vi "VNA Empty Driver Output.vi"() -> (0 "VNA Driver Output":T1 {"Parameters Measured"."Channel" min=1 max=99 step=1; "Parameters Measured"."Parameter"."Stimulus Port" min=1 step=1; "Parameters Measured"."Parameter"."Response Port" min=1 step=1})   [LabVIEW 2011]
uses:
  tests/S Parameter/TypeDefs/SP Parameter.ctl
  tests/S Parameter/TypeDefs/SP Calibration State.ctl
  VNA Measurement Format.ctl
  VNA Parameter to Measure.ctl
  VNA Driver Ref.ctl
  tests/S Parameter/TypeDefs/SP Data.ctl
  VNA Driver Output.ctl
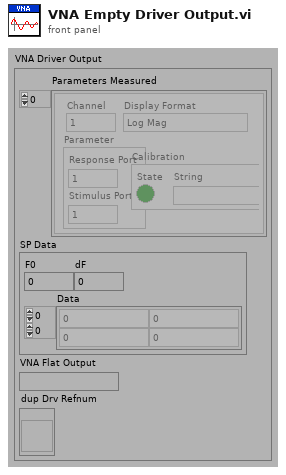
[diagram p1: front panel]
types:
  T1 = typedef "VNA Driver Output.ctl" = cluster{"Parameters Measured":T2[], "SP Data":T6, "VNA Flat Output":string, "dup Drv Refnum":T7}
  T2 = typedef "VNA Parameter to Measure.ctl" = cluster{"Channel":i8, "Parameter":T3, "Calibration":T4, "Display Format":T5}
  T3 = typedef "SP Parameter.ctl" = cluster{"Stimulus Port":i8, "Response Port":i8}
  T4 = typedef "SP Calibration State.ctl" = cluster{"State":bool, "String":string}
  T5 = typedef "VNA Measurement Format.ctl" = enum32{"Log Mag", "Phase", "Delay", "Smith (R+jX)", "Polar (Re/Im)", "Linear Mag", "SWR", "Real", "Imaginary", "Smith (Lin/Phase)", "Smith (Log/Phase)", "Smith (Real/Imag)", "Smith (G+jB)", "Polar (Lin)", "Polar (Log)", "Expanded Phase", "Positive Phase", "Inverted Smith", "Unwrapped Phase", "Power Out"}
  T6 = typedef "SP Data.ctl" = cluster{"F0":dbl, "dF":dbl, "Data":cdb[][]}
  T7 = typedef "VNA Driver Ref.ctl" = refnum<vi>
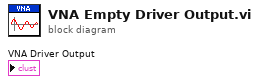
[diagram p0: block diagram]
diagram:
